vi "Write Parcel pickup address.vi"(8 "error in (no error)":errorcluster, 10 "Parcel pickup address":string, 11 "Delivery in":refnum<class "Delivery.lvclass">) -> (0 "error out":errorcluster, 3 "Delivery out":refnum<class "Delivery.lvclass">)   [LabVIEW 2019, in "Delivery.lvclass"]
uses:
  Delivery.lvclass
  Delivery.lvclass/Delivery.ctl
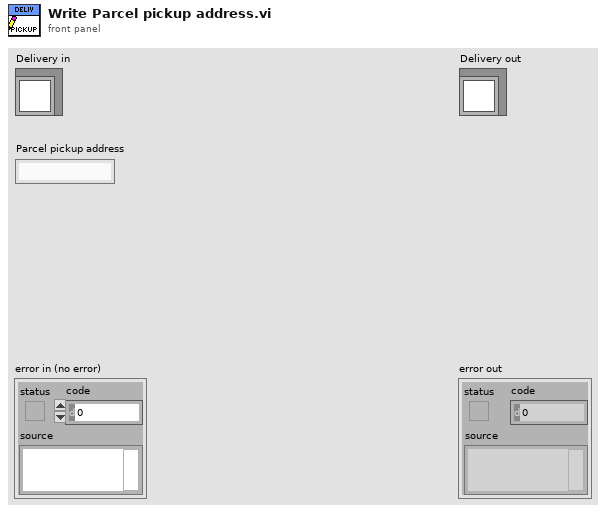
[diagram p1: front panel]
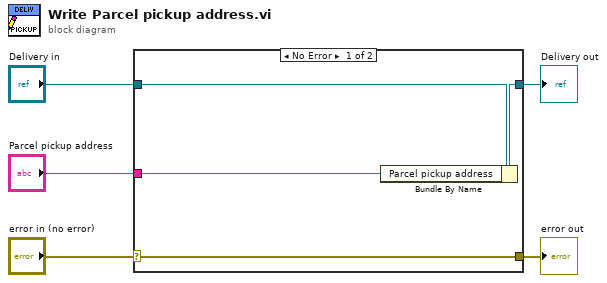
[diagram p0: block diagram]
diagram:
  n1 = case shown="No Error" "error in (no error)" {
    selector: "error in (no error)" -> [w9 w10]
    tunnel: [w9 w10] -> w4
    tunnel: [w7 w11] -> w2
    tunnel: "Delivery in" -> [w8 w11]
    tunnel: "Parcel pickup address" -> [w6 _]
    frame No Error {
      n2 = Bundle By Name(cluster=w8, "Parcel pickup address"=w6) -> (w7:refnum<class "Delivery.lvclass">)
    }
    frame Error {
    }
  }
  "error out" <- w4
  "Delivery out" <- w2
